vi "Main.vi"() -> ()   [LabVIEW 2014]
uses:
  <vilib>/Utility/miscctls.llb/LVPoint32TypeDef.ctl
  <vilib>/Utility/miscctls.llb/LVRowAndColumnTypeDef.ctl
panel:
  in  "Active Cell:Cell Background Color":u32
  out "Active Cell:Active Cell":T1
  in  "channels 2":i32(listbox)
  out "Cell Position":T1
  out "PlatMods":T2
  out "Mods":cluster{"Double Click":bool, "Menu Key":bool}
  out "Button":u16
  out "Coords":T3
  in  "stop":bool
  in  "Remove Button":bool
  in  "Add Button":bool
  in  "channels":i32(listbox)
  in  "settings":bool
  in  "Import":bool
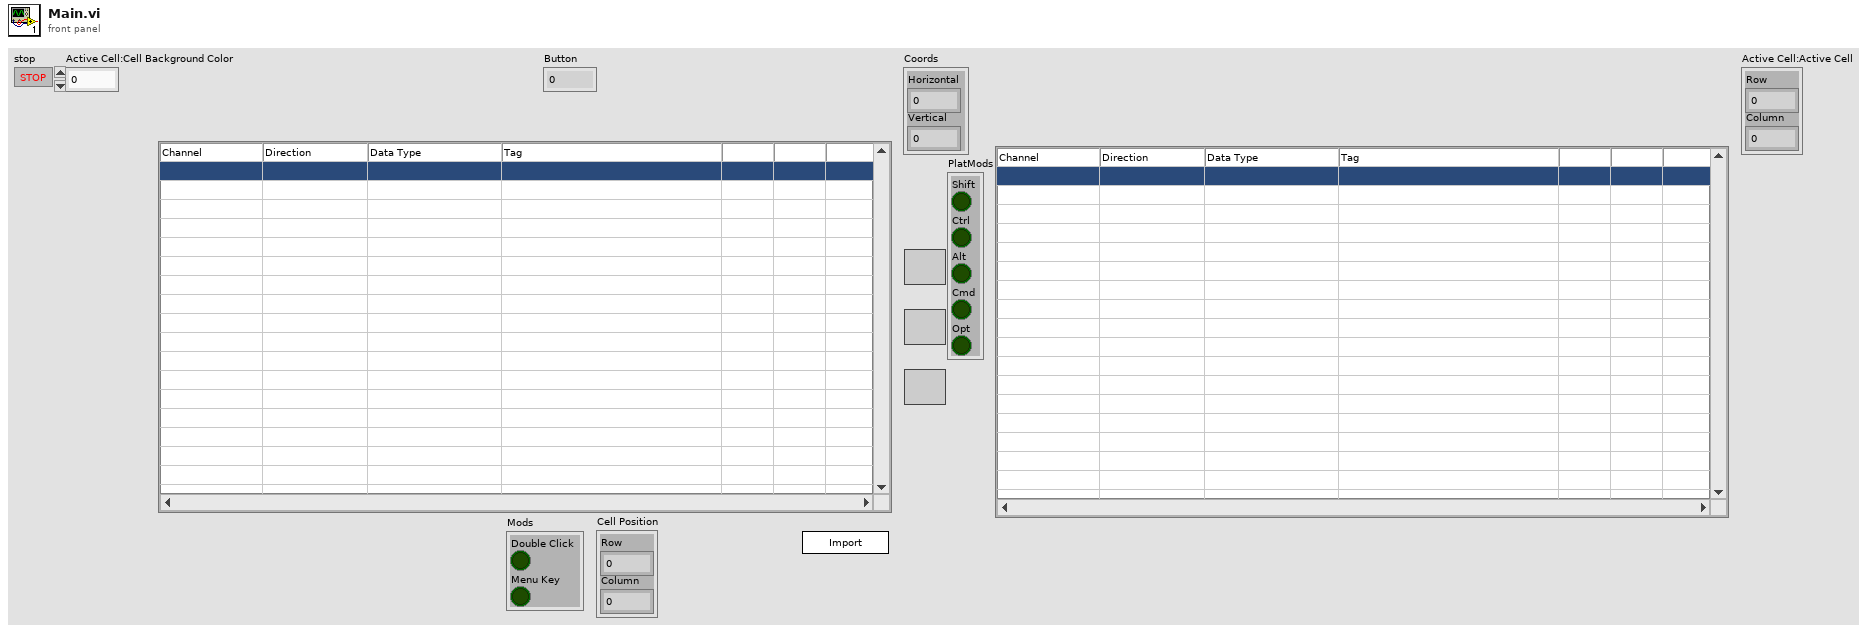
[diagram p1: front panel]
types:
  T1 = typedef "LVRowAndColumnTypeDef.ctl" = cluster{"Row":i32, "Column":i32}
  T2 = cluster{"Shift":bool, "Ctrl":bool, "Alt":bool, "Cmd":bool, "Opt":bool}
  T3 = typedef "LVPoint32TypeDef.ctl" = cluster{"Horizontal":i32, "Vertical":i32}
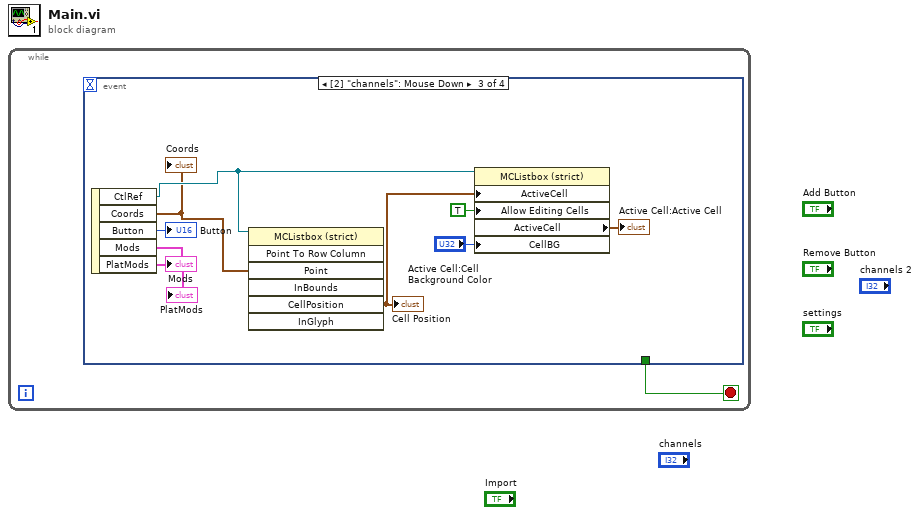
[diagram p0: block diagram]
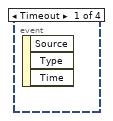
[diagram p2: hidden frame]
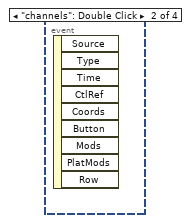
[diagram p3: hidden frame]
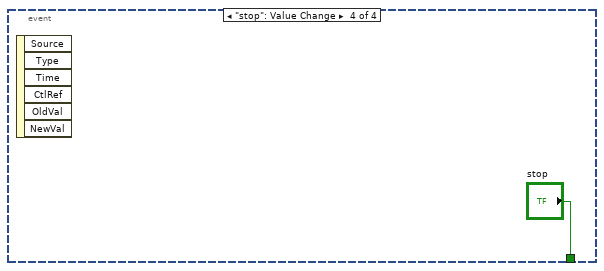
[diagram p4: hidden frame]
diagram:
  n1 = while {
    stop <- w1 stop-if-true
    n2 = event shown="[2] \"channels\": Mouse Down" {
      selector: _ -> [_ _ _ _]
      dyn-events: _ -> [_ _ _ _]
      timeout: _ -> [_ _ _ _]
      tunnel: [_ _ _ "stop"] -> w1
      event Timeout {
        n3 = event-data() -> ()  [unwired: 1 in, 3 out]
      }
      event "channels": Double Click {
        n4 = event-data() -> ()  [unwired: 1 in, 9 out]
      }
      event "channels": Mouse Down {
        n5 = event-data() -> ("CtlRef"=w7:refnum<vi>, "Coords"=w6:T3, "Button"=→"Button":u16, "Mods"=→"Mods":cluster{"Double Click":bool, "Menu Key":bool}, "PlatMods"=→"PlatMods":T2)  [unwired: 1 in]
        "Coords" <- w6
        n6 = invoke class="MCListbox (strict)" method="Point To Row Column"(reference=w7, "Point"=w6) -> ("CellPosition"=w5:T1)  [unwired: 5 in, 6 out]
        "Cell Position" <- w5
        n7 = property class="MCListbox (strict)"(reference=w7, "ActiveCell"=w5, "Allow Editing Cells"=TRUE, "CellBG"="Active Cell:Cell Background Color") -> ("ActiveCell"=→"Active Cell:Active Cell":T1)  [unwired: 1 in, 2 out]
      }
      event "stop": Value Change {
        n8 = event-data() -> ()  [unwired: 1 in, 6 out]
      }
    }
  }
